vi "Convert Input Terminal Cfg to DAQmx Style.vi"(11 "input terminal cfg":T1 caption="Data justification") -> (3 "DAQmx input terminal cfg":i32(ring)=10106 items=["Default"=-1, "RSE"=10083, "NRSE"=10078, "Differential"=10106, "Pseudodifferential"=12529])   [LabVIEW 2021, in "DAQmx utility.lvlib"]
uses:
  DAQmx utility.lvlib
  input terminal configuration.ctl
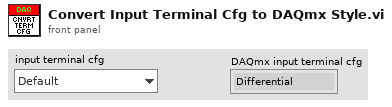
[diagram p1: front panel]
types:
  T1 = typedef "DAQmx utility.lvlib/input terminal configuration.ctl" = enum32{"Default", "NRSE", "RSE", "Differential", "Pseudodifferential"}
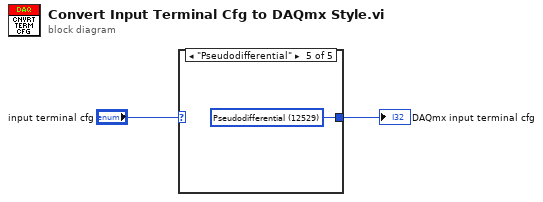
[diagram p0: block diagram]
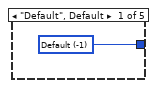
[diagram p2: hidden frame]
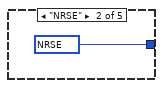
[diagram p3: hidden frame]
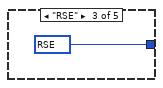
[diagram p4: hidden frame]
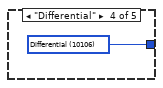
[diagram p5: hidden frame]
diagram:
  n1 = case shown="\"Pseudodifferential\"" "input terminal cfg" {
    tunnel: [w3 w4 w5 w6 w7] -> w1
    frame "Default", Default {
      w3 = -1 items=["Default"=-1, "RSE"=10083, "NRSE"=10078, "Differential"=10106, "Pseudodifferential"=12529] ("input terminal configuration")
    }
    frame "NRSE" {
      w4 = 10078 items=["Default"=-1, "RSE"=10083, "NRSE"=10078, "Differential"=10106, "Pseudodifferential"=12529] ("input terminal configuration")
    }
    frame "RSE" {
      w5 = 10083 items=["Default"=-1, "RSE"=10083, "NRSE"=10078, "Differential"=10106, "Pseudodifferential"=12529] ("input terminal configuration")
    }
    frame "Differential" {
      w6 = 10106 items=["Default"=-1, "RSE"=10083, "NRSE"=10078, "Differential"=10106, "Pseudodifferential"=12529] ("input terminal configuration")
    }
    frame "Pseudodifferential" {
      w7 = 12529 items=["Default"=-1, "RSE"=10083, "NRSE"=10078, "Differential"=10106, "Pseudodifferential"=12529] ("input terminal configuration")
    }
  }
  "DAQmx input terminal cfg" <- w1
